vi "sound.vi"(0 "Sound File":path) -> ()   [LabVIEW 2014]
uses:
  globals/AzCamGlobals.vi
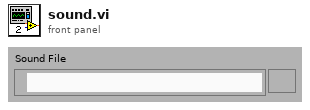
[diagram p1: front panel]
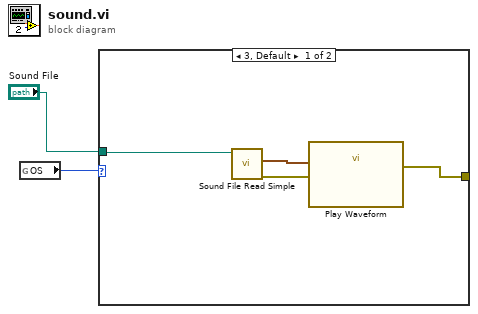
[diagram p0: block diagram]
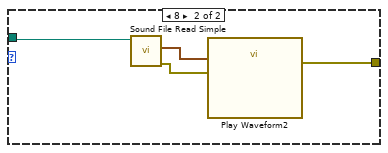
[diagram p2: hidden frame]
diagram:
  n1 = global read "AzCamGlobals.vi" "OS"() -> (w1:i32)
  n2 = case shown="3, Default" w1 {
    tunnel: "Sound File" -> [w6 w9]
    tunnel: [w3 w7] -> _
    frame 3, Default {
      n3 = call <vilib>:"Sound File Read Simple.vi"("path"=w6) -> ("error out"=w4:errorcluster, "data"=w5:waveform(dbl)[])  [unwired: 7 in, 2 out]
      n4 = call "Play Waveform"("Data"=w5, "error in"=w4) -> ("error out"=w3:errorcluster)  [unwired: 17 in]
    }
    frame 8 {
      n5 = call <vilib>:"Sound File Read Simple.vi"("path"=w9) -> ("error out"=w8:errorcluster, "data"=w10:waveform(dbl)[])  [unwired: 7 in, 2 out]
      n6 = call "Play Waveform2"("Data"=w10, "error in"=w8) -> ("error out"=w7:errorcluster)  [unwired: 17 in]
    }
  }
